vi "Test World To Local.vi"(11 "Test Case In":refnum<class "Utility.lvclass">) -> (0 "error out":errorcluster, 3 "Test Case Out":refnum<class "Utility.lvclass">)   [LabVIEW 2021, in "Utility.lvclass"]
uses:
  Utility.lvclass
  C:/Program Files (x86)/National Instruments/LabVIEW 2026/vi.lib/Astemes/LUnit/Test Case.lvclass
  <vilib>/Astemes/LUnit/Test Case.lvclass/Test Case.ctl
  4993e8ee-a06a-463a-9684-69129f64d5ce.vi
  Re-use Libraries/Vector 2D/Vector 2D.lvclass
  302ad57d-a235-4a34-ad65-6d5892710abb.vi
  <vilib>/Astemes/LUnit/Test Case.lvclass
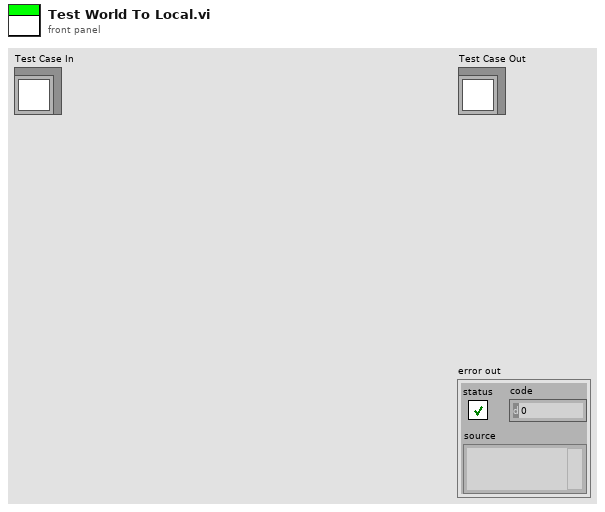
[diagram p1: front panel]
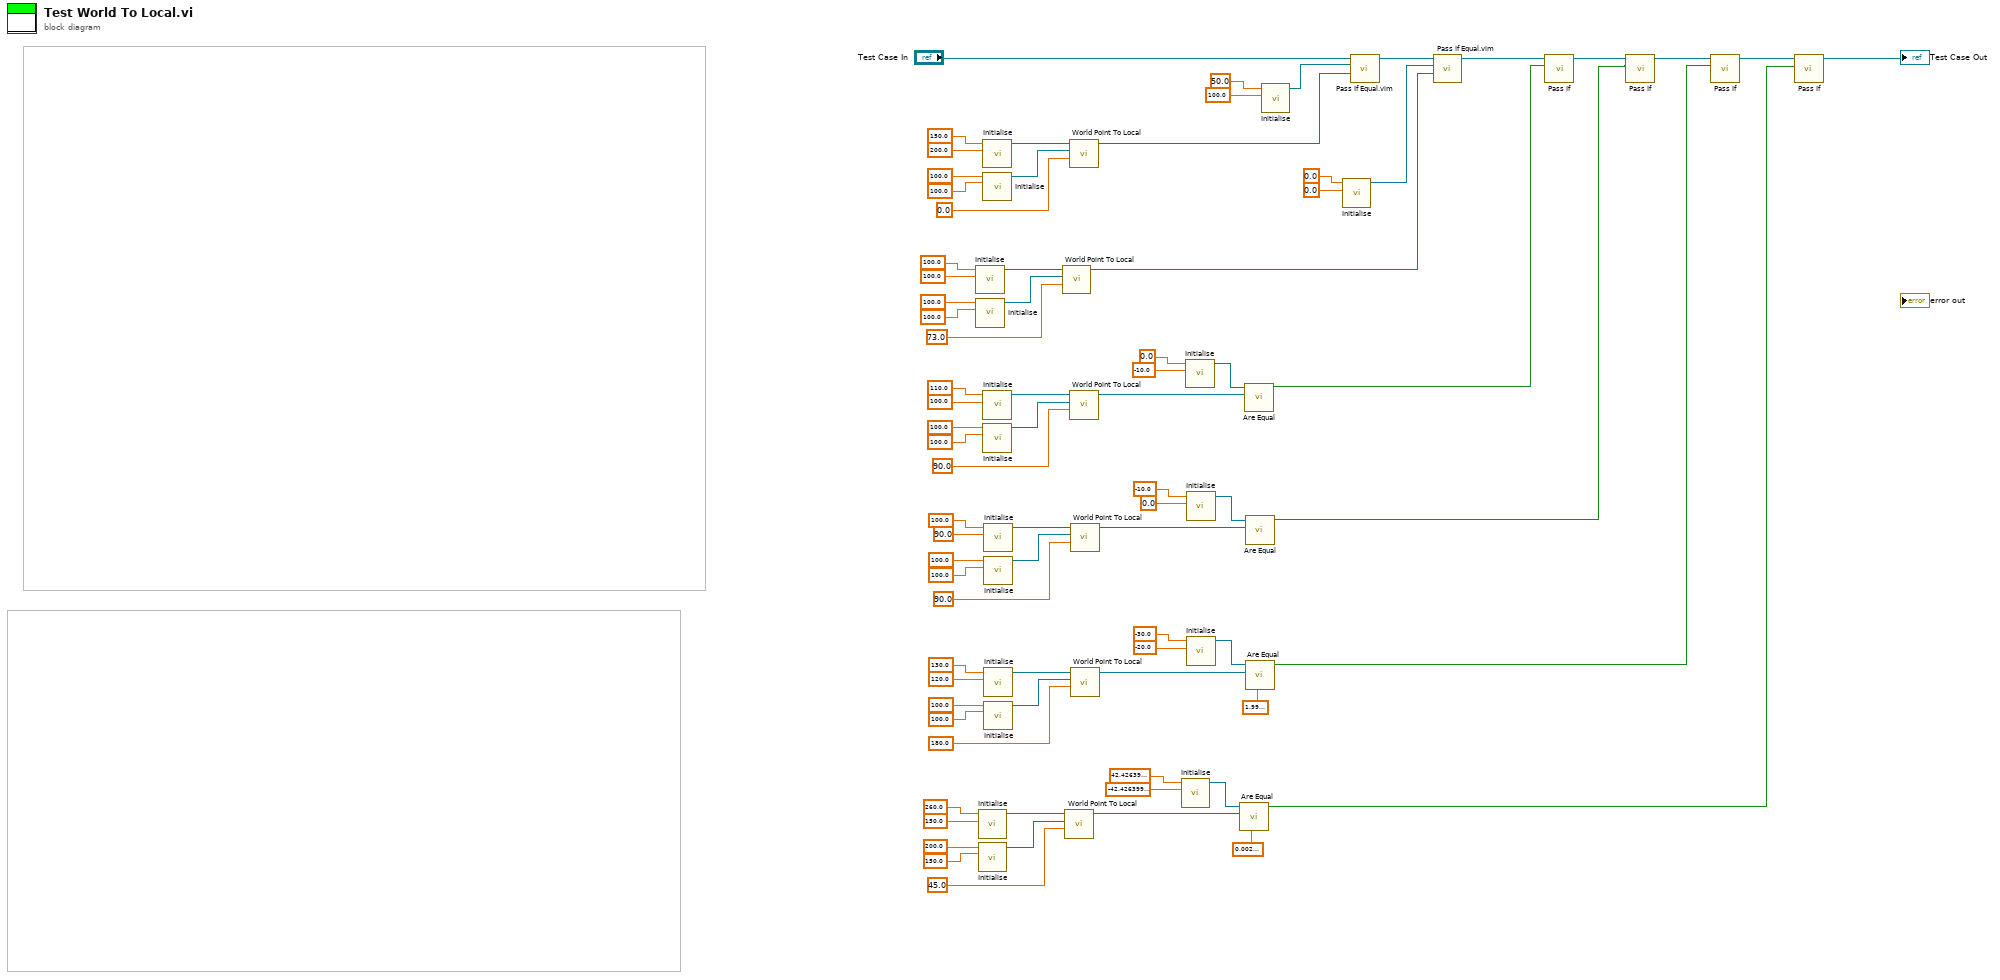
[diagram p0: block diagram]
diagram:
  n1 = call "Initialise.vi"("y"=sgl 100.0, "x"=sgl 100.0) -> ("Vector 2D out"=w61:refnum<class "Vector 2D.lvclass">)  [unwired: 9 in]
  n2 = call "Initialise.vi"("y"=sgl 100.0 ("x"), "x"=sgl 100.0) -> ("Vector 2D out"=w62:refnum<class "Vector 2D.lvclass">)  [unwired: 9 in]
  n3 = call "Initialise.vi"("y"=sgl 150.0, "x"=sgl 260.0) -> ("Vector 2D out"=w4:refnum<class "Vector 2D.lvclass">)  [unwired: 9 in]
  n4 = call "Initialise.vi"("y"=sgl 150.0 ("x"), "x"=sgl 200.0) -> ("Vector 2D out"=w5:refnum<class "Vector 2D.lvclass">)  [unwired: 9 in]
  n5 = call "Initialise.vi"("y"=sgl 200.0, "x"=sgl 150.0) -> ("Vector 2D out"=w78:refnum<class "Vector 2D.lvclass">)  [unwired: 9 in]
  n6 = call "Initialise.vi"("y"=sgl 100.0 ("x"), "x"=sgl 100.0) -> ("Vector 2D out"=w77:refnum<class "Vector 2D.lvclass">)  [unwired: 9 in]
  n7 = call "Initialise.vi"("y"=sgl 100.0, "x"=sgl 110.0) -> ("Vector 2D out"=w55:refnum<class "Vector 2D.lvclass">)  [unwired: 9 in]
  n8 = call "Initialise.vi"("y"=sgl 100.0 ("x"), "x"=sgl 100.0) -> ("Vector 2D out"=w54:refnum<class "Vector 2D.lvclass">)  [unwired: 9 in]
  n9 = call "Initialise.vi"("y"=sgl 90.0, "x"=sgl 100.0) -> ("Vector 2D out"=w32:refnum<class "Vector 2D.lvclass">)  [unwired: 9 in]
  n10 = call "Initialise.vi"("y"=sgl 100.0 ("x"), "x"=sgl 100.0) -> ("Vector 2D out"=w33:refnum<class "Vector 2D.lvclass">)  [unwired: 9 in]
  n11 = call "Initialise.vi"("y"=sgl 120.0, "x"=sgl 130.0) -> ("Vector 2D out"=w29:refnum<class "Vector 2D.lvclass">)  [unwired: 9 in]
  n12 = call "Initialise.vi"("y"=sgl 100.0 ("x"), "x"=sgl 100.0) -> ("Vector 2D out"=w28:refnum<class "Vector 2D.lvclass">)  [unwired: 9 in]
  n13 = call "World Point To Local.vi"("Rotation [deg]"=sgl 73.0, "Sprite Center"=w62, "World Point"=w61) -> ("Local Point"=w56:refnum<class "Vector 2D.lvclass">)  [unwired: 8 in]
  n14 = call "World Point To Local.vi"("Rotation [deg]"=sgl 45.0, "Sprite Center"=w5, "World Point"=w4) -> ("Local Point"=w14:refnum<class "Vector 2D.lvclass">)  [unwired: 8 in]
  n15 = call "World Point To Local.vi"("Rotation [deg]"=sgl 0.0, "Sprite Center"=w77, "World Point"=w78) -> ("Local Point"=w69:refnum<class "Vector 2D.lvclass">)  [unwired: 8 in]
  n16 = call "World Point To Local.vi"("Rotation [deg]"=sgl 90.0, "Sprite Center"=w54, "World Point"=w55) -> ("Local Point"=w45:refnum<class "Vector 2D.lvclass">)  [unwired: 8 in]
  n17 = call "World Point To Local.vi"("Rotation [deg]"=sgl 90.0, "Sprite Center"=w33, "World Point"=w32) -> ("Local Point"=w42:refnum<class "Vector 2D.lvclass">)  [unwired: 8 in]
  n18 = call "World Point To Local.vi"("Rotation [deg]"=sgl 180.0, "Sprite Center"=w28, "World Point"=w29) -> ("Local Point"=w19:refnum<class "Vector 2D.lvclass">)  [unwired: 8 in]
  n19 = call "Initialise.vi"("y"=sgl -42.4264, "x"=sgl 42.4264) -> ("Vector 2D out"=w13:refnum<class "Vector 2D.lvclass">)  [unwired: 9 in]
  n20 = call "Initialise.vi"("y"=sgl -10.0, "x"=sgl 0.0) -> ("Vector 2D out"=w46:refnum<class "Vector 2D.lvclass">)  [unwired: 9 in]
  n21 = call "Initialise.vi"("y"=sgl 0.0, "x"=sgl -10.0) -> ("Vector 2D out"=w41:refnum<class "Vector 2D.lvclass">)  [unwired: 9 in]
  n22 = call "Initialise.vi"("y"=sgl -20.0, "x"=sgl -30.0) -> ("Vector 2D out"=w20:refnum<class "Vector 2D.lvclass">)  [unwired: 9 in]
  n23 = call "Are Equal.vi"("Tolerance"=sgl 0.002, "Vector 2"=w14, "Vector 1"=w13) -> ("Equal"=w1:bool)  [unwired: 8 in]
  n24 = call "Are Equal.vi"("Vector 2"=w45, "Vector 1"=w46) -> ("Equal"=w43:bool)  [unwired: 9 in]
  n25 = call "Are Equal.vi"("Vector 2"=w42, "Vector 1"=w41) -> ("Equal"=w30:bool)  [unwired: 9 in]
  n26 = call "Are Equal.vi"("Tolerance"=sgl 2e-06, "Vector 2"=w19, "Vector 1"=w20) -> ("Equal"=w17:bool)  [unwired: 8 in]
  n27 = call "Initialise.vi"("y"=sgl 100.0, "x"=sgl 50.0) -> ("Vector 2D out"=w68:refnum<class "Vector 2D.lvclass">)  [unwired: 9 in]
  n28 = call "Initialise.vi"("y"=sgl 0.0, "x"=sgl 0.0) -> ("Vector 2D out"=w57:refnum<class "Vector 2D.lvclass">)  [unwired: 9 in]
  n29 = call "Pass If Equal.vim"("Actual"=w69, "Expected"=w68, "LUnit Test Case In"="Test Case In") -> ("LUnit Test Case Out"=w60:refnum<class "Utility.lvclass">)  [unwired: 7 in, 1 out]
  n30 = call "Pass If Equal.vim"("Actual"=w56, "Expected"=w57, "LUnit Test Case In"=w60) -> ("LUnit Test Case Out"=w44:refnum<class "Utility.lvclass">)  [unwired: 7 in, 1 out]
  n31 = call <vilib>:"Pass If.vi"("Pass?"=w43, "LUnit Test Case In"=w44) -> ("LUnit Test Case Out"=w31:refnum<class "Utility.lvclass">)  [unwired: 8 in, 1 out]
  n32 = call <vilib>:"Pass If.vi"("Pass?"=w30, "LUnit Test Case In"=w31) -> ("LUnit Test Case Out"=w18:refnum<class "Utility.lvclass">)  [unwired: 8 in, 1 out]
  n33 = call <vilib>:"Pass If.vi"("Pass?"=w17, "LUnit Test Case In"=w18) -> ("LUnit Test Case Out"=w3:refnum<class "Utility.lvclass">)  [unwired: 8 in, 1 out]
  n34 = call <vilib>:"Pass If.vi"("Pass?"=w1, "LUnit Test Case In"=w3) -> ("LUnit Test Case Out"=→"Test Case Out":refnum<class "Utility.lvclass">)  [unwired: 8 in, 1 out]
